vi "lookuptable(for_secondNM)_0921.vi"(5 "data of 5th order formula\nts,tair,a1-a6 \n(input from the first NM)":dbl[](array[numeric]), 7 "step count NM":dbl, 11 "buffer ratio":dbl) -> (6 "output cluster 2":T1, 10 "time180":dbl, 12 "reset step(indicator)":bool, 13 "start to calculate the power":bool, 14 "start to calculate the cost":bool, 15 "period":dbl)   [LabVIEW 2019]
panel:
  in  "reset step":bool
  out "p_final":dbl
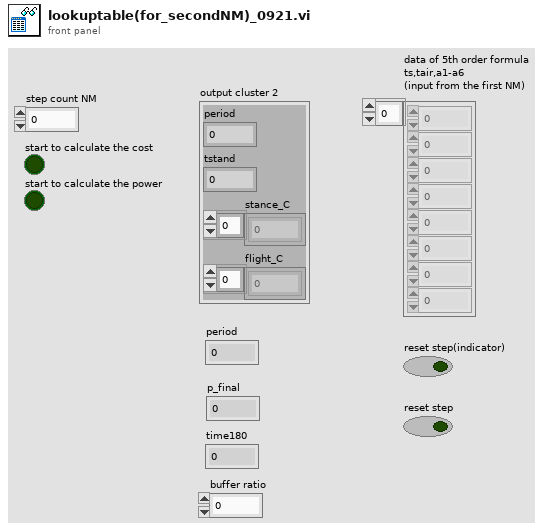
[diagram p1: front panel]
types:
  T1 = cluster{"period":dbl, "tstand":dbl, "stance_C":dbl[], "flight_C":dbl[]}
  T2 = cluster{"Numeric":dbl, "Numeric":dbl, "Numeric":dbl, "Numeric":dbl, "Numeric":dbl, "Numeric":dbl, "Numeric":dbl, "Numeric":dbl}
  T3 = cluster{"pf":dbl, "vf":dbl, dbl, "Numeric":dbl, "Numeric":dbl, "buffer ratio":dbl}
  T4 = cluster{dbl, "Numeric":dbl, dbl[], "flight_C":dbl[]}
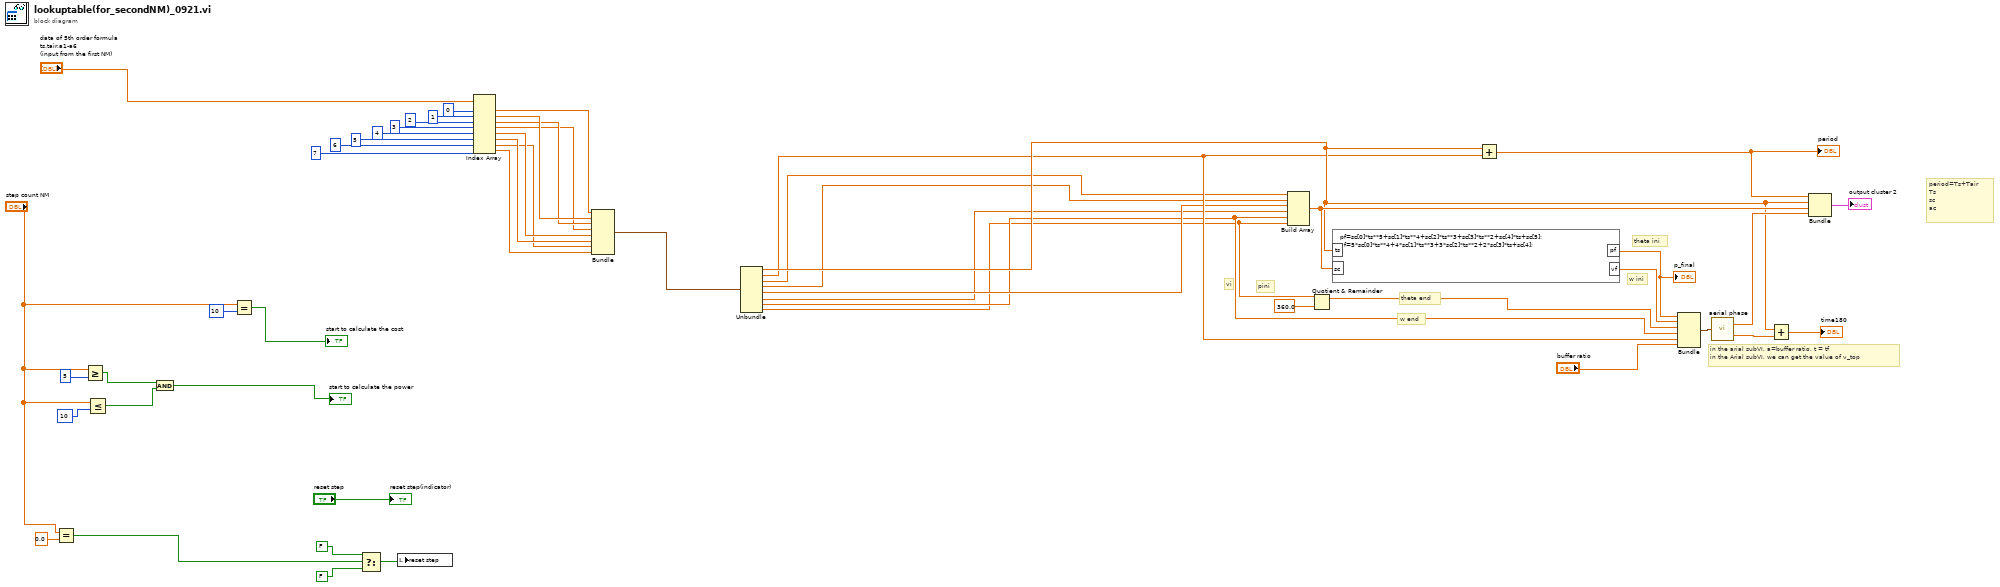
[diagram p0: block diagram]
diagram:
  # "in the arial subVI, a=buffer ratio, t = tf\nin the Arial subVI, we can get the value of v_top"
  # "period=Ts+Tair\nTs\nsc\nac"
  # "w ini"
  # "theta ini"
  # "w end"
  # "theta end"
  # "vi"
  # "pini"
  n1 = Equal?(x="step count NM", y=0.0) -> (x = y?=w7:bool)
  n2 = Greater Or Equal?(x="step count NM", y=5) -> (x >= y?=w4:bool)
  n3 = Less Or Equal?(x="step count NM", y=10) -> (x <= y?=w3:bool)
  n4 = And(x=w4, y=w3) -> (x .and. y?=→"start to calculate the power":bool)
  n5 = Equal?(x="step count NM", y=10) -> (x = y?=→"start to calculate the cost":bool)
  n6 = Select(t=FALSE, s=w7, f=FALSE) -> (s? t:f=w12:bool)
  n7 = local write "reset step"(w12) -> ()
  n8 = Index Array(array="data of 5th order formula\nts,tair,a1-a6 \n(input from the first NM)", index #1=0 ("index"), index #2=1 ("index"), index #3=2 ("index"), index #4=3 ("index"), index #5=4 ("index"), index #6=5 ("index"), index #7=6 ("index"), index #8=7 ("index")) -> (element #1=w33:dbl, element #2=w40:dbl, element #3=w39:dbl, element #4=w38:dbl, element #5=w37:dbl, element #6=w36:dbl, element #7=w35:dbl, element #8=w34:dbl)
  n9 = Bundle("Numeric"=w33, "Numeric"=w40, "Numeric"=w39, "Numeric"=w38, "Numeric"=w37, "Numeric"=w36, "Numeric"=w35, "Numeric"=w34) -> (w15:T2)  [unwired: 1 in]
  n10 = Unbundle(w15) -> ("Numeric"=w24:dbl, "Numeric"=w23:dbl, "Numeric"=w22:dbl, "Numeric"=w21:dbl, "Numeric"=w20:dbl, "Numeric"=w19:dbl, "Numeric"=w18:dbl, "Numeric"=w17:dbl)
  n11 = Build Array(w22, w21, w20, w19, w18, w17) -> (w45:dbl[])
  n12 = Quotient & Remainder(x=w17, y=360.0) -> (x-y*floor(x/y)=w41:dbl)  [unwired: 1 out]
  n13 = formula code="pf=sc[0]*ts**5+sc[1]*ts**4+sc[2]*ts**3+sc[3]*ts**2+sc[4]*ts+sc[5];\nvf=5*sc[0]*ts**4+4*sc[1]*ts**3+3*sc[2]*ts**2+2*sc[3]*ts+sc[4];"("sc"=w45, "ts"=w24) -> ("pf"=w49:dbl, "vf"=w43:dbl)
  "p_final" <- w49
  n14 = Add(x=w24, y=w23) -> (x+y=w46:dbl)
  "period" <- w46
  n15 = Bundle("pf"=w49, "vf"=w43, w41, "Numeric"=w18, "Numeric"=w23, "buffer ratio"="buffer ratio") -> (w48:T3)  [unwired: 1 out]
  n16 = call "aerial phase.vi"("aerial condition"=w48) -> ("time180"=w47:dbl, "flight_C"=w44:dbl[])  [unwired: 2 in]
  n17 = Add(x=w24, y=w47) -> (x+y=→"time180":dbl)
  n18 = Bundle(w46, "Numeric"=w24, w45, "flight_C"=w44) -> (→"output cluster 2":T4)  [unwired: 1 in]
  "reset step(indicator)" <- "reset step"
